vi "Player Name.vi"() -> (2 "Name":string)   [LabVIEW 2020, in "NonOOPlayer.lvlib"]
uses:
  NonOOPlayer.lvlib
panel:
  # "Edit the contents of the string constant on the block diagram to set the name for your AI player."
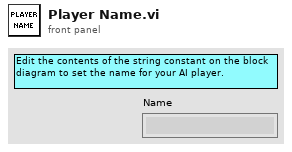
[diagram p1: front panel]
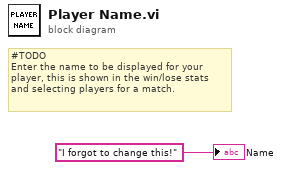
[diagram p0: block diagram]
diagram:
  # "#TODO\nEnter the name to be displayed for your player, this is shown in the win/lose stats and selecting players for a match."
  "Name" <- "I forgot to change this!" ("Name")
